vi "VideoTest.vi"() -> ()   [LabVIEW 2014]
uses:
  <vilib>/vision/NI_Vision_Development_Module.lvlib
panel:
  in  "BCG Values":T1={"Brightness"=128.0, "Contrast"=45.0, "Gamma"=1.0} {"Brightness" min=0 max=255 step=1 format="%.2f"; "Contrast" min=1 max=89 step=1 format="%.2f"; "Gamma" min=0.1 max=10 step=0.01 format="%.2f"}
  in  "stop":bool
  in  "Black Level":dbl min=0.0 max=511.0
  in  "Black Level Selector":u32(ring) items=["Analog"]
  in  "Gain (Raw)":i64 min=0 max=384 step=1
  in  "Gain":dbl=1.0 min=1.0 max=4.0
  in  "Gain Selector":u32(ring) items=["Sensor", "Digital"]
  in  "Exposure Time":dbl=41000.0 min=61.0 max=16000000.0
  out "Image Out":T2(plugin-control)
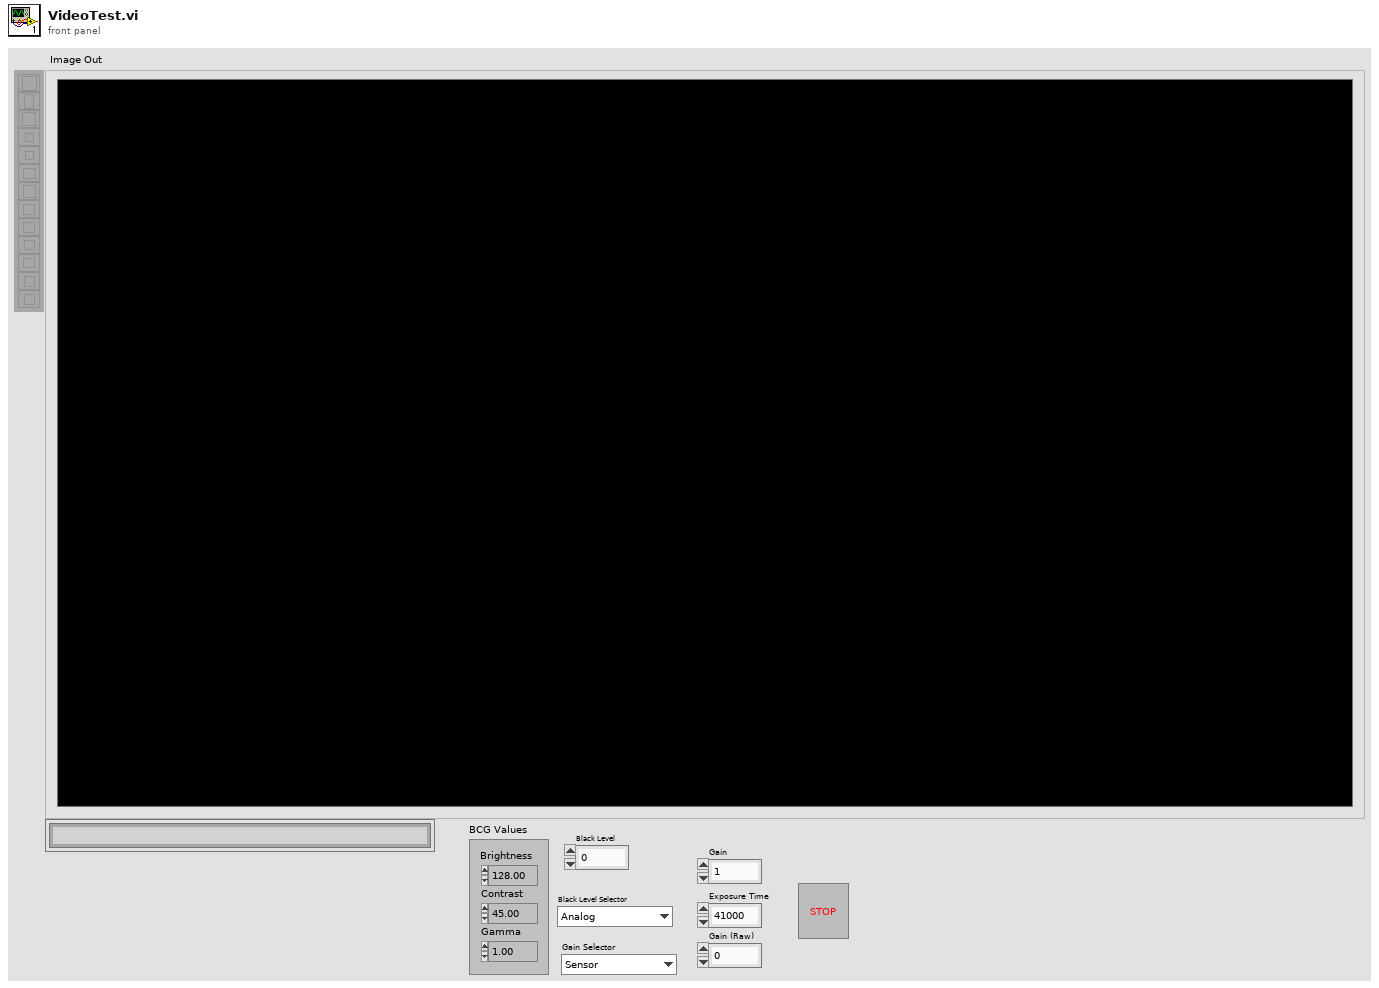
[diagram p1: front panel]
types:
  T1 = cluster{"Brightness":sgl, "Contrast":sgl, "Gamma":sgl}
  T2 = typedef "IMAQ Image.ctl" = refnum<image>
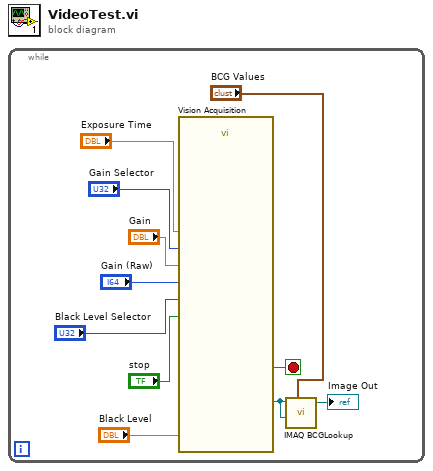
[diagram p0: block diagram]
diagram:
  n1 = while {
    stop <- w11 stop-if-true
    n2 = call "Vision Acquisition"("Exposure Time"="Exposure Time", "Gain Selector"="Gain Selector", "Gain"="Gain", "Gain (Raw)"="Gain (Raw)", "Black Level Selector"="Black Level Selector", "Stop (F)"="stop", "Black Level"="Black Level") -> ("Image Out"=w2:T2, "Stopped"=w11:bool)  [unwired: 16 in, 3 out]
    n3 = call "IMAQ BCGLookup"("Image Src"=w2, "BCG Values"="BCG Values", "Image Dst"=w2) -> ("Image Dst Out"=→"Image Out":T2)  [unwired: 4 in, 1 out]
  }
